vi "ajouterdonneetache.vi"(0 "Req":string caption="heure", 1 "Deb":string caption="heure", 2 "Statut":string caption="heure", 3 "Debut":string caption="heure", 4 "Fin":string caption="heure", 5 "Name":string, 6 "Fichier DB":string) -> ()   [LabVIEW 2024]
uses:
  <vilib>/drjdpowell/SQLite Library/SQL Connection/Open (string).vi
  <vilib>/drjdpowell/SQLite Library/SQL Connection/Execute SQL (No results).vi
  <vilib>/drjdpowell/SQLite Library/SQL Connection/Connection.lvclass
  <vilib>/drjdpowell/SQLite Library/SQLite.lvlib
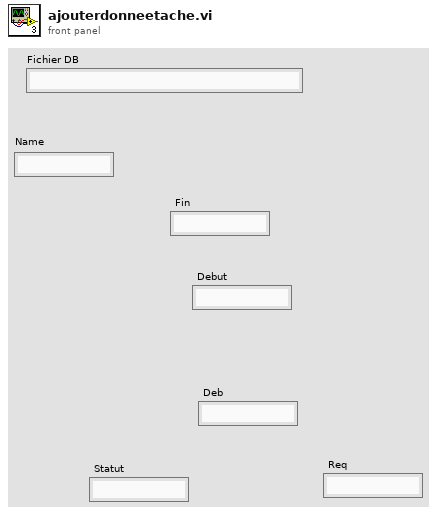
[diagram p1: front panel]
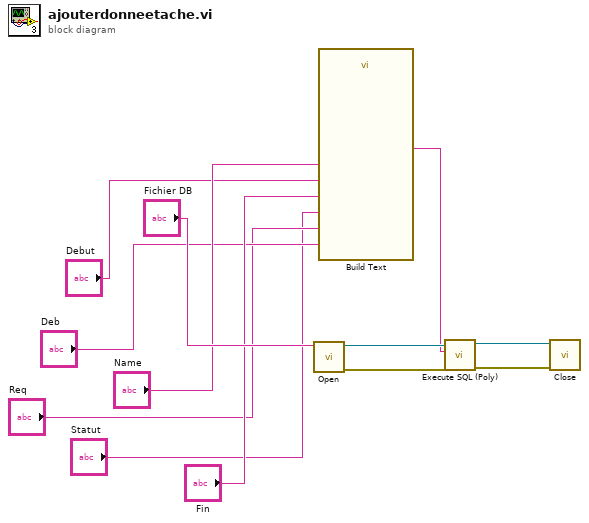
[diagram p0: block diagram]
diagram:
  n1 = call-poly <vilib>:"Open.vi"("db file"="Fichier DB") -> ("error out"=w11:errorcluster, "SQLite Connection"=w12:refnum<class "Connection.lvclass">)  [unwired: 9 in]
  n2 = call "Build Text"("statut"="Statut", "deb"="Deb", "name"="Name", "debut"="Debut", "fin"="Fin", "req"="Req") -> ("Result"=w10:string)  [unwired: 8 in, 1 out]
  n3 = call-poly <vilib>:"Execute SQL (Poly).vi"("error in (no error)"=w11, "SQL"=w10, "SQLite Connection in"=w12) -> ("error out"=w9:errorcluster, "SQLite Connection"=w8:refnum<class "Connection.lvclass">)  [unwired: 7 in]
  n4 = call-dynamic "Close.vi"("error in (no error)"=w9, "SQLite Connection in"=w8) -> ()  [unwired: 9 in, 1 out]
